vi "test2.vi"() -> ()   [LabVIEW 2010]
panel:
  in  "Stopp":bool
  out "Numerisch":i32
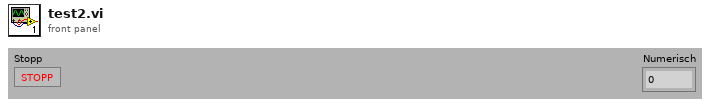
[diagram p1: front panel]
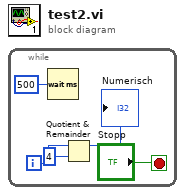
[diagram p0: block diagram]
diagram:
  n1 = while {
    i -> [w4]
    stop <- "Stopp" stop-if-true
    n2 = Wait (ms)(milliseconds to wait=u32 500 ("Zu wartende ms")) -> ()  [unwired: 1 out]
    n3 = Quotient & Remainder(x=w4, y=4) -> (x-y*floor(x/y)=→"Numerisch":i32)  [unwired: 1 out]
  }
